vi "Instr_InitObject.vi"(8 "error in (no error)":errorcluster, 9 "Instrument Configuration":variant, 10 "GPIB address":string, 11 "KE236 in":refnum<class "KE236.lvclass">) -> (0 "error out":errorcluster, 3 "KE236 out":refnum<class "KE236.lvclass">)   [LabVIEW 2013, in "KE236.lvclass"]
uses:
  KE236.lvclass
  SupplyControl.lvclass
  InstrumentSetup.vi
  KE236_CommandsGlobal.vi
  InstrControl.lvclass
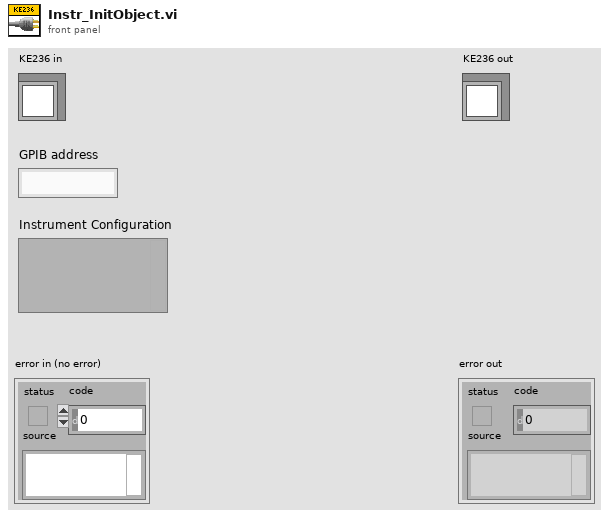
[diagram p1: front panel]
types:
  T1 = cluster{"current \ncompliance level":dbl, "compliance/\nmeasurement range (auto:0)":u16, "KE236":refnum<class "KE236.lvclass">}
  T2 = cluster{"Instrument name":string, "Command \"Reset\"":string, "Command \"Initialise\"":string, "Command \"Arm\"":string, "Command \"SetVolts\"":string, "Command \"Compliance?\"":string, "Command \"Standby\"":string, "Command \"Read Current\"":string}
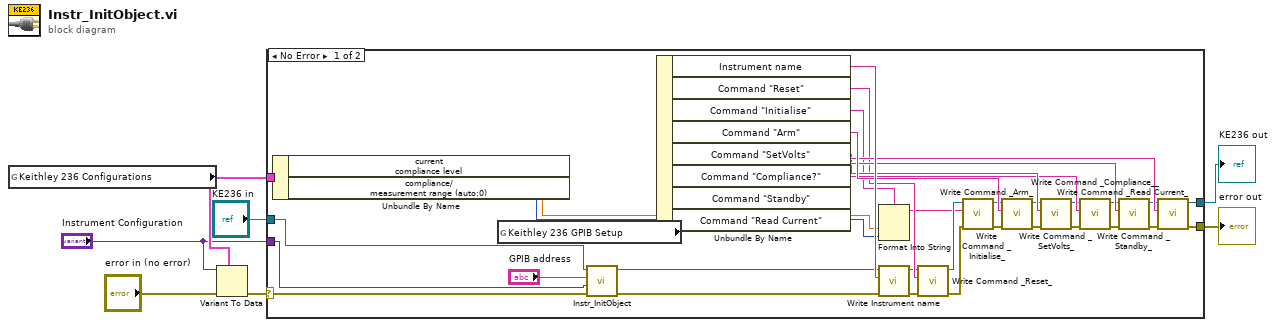
[diagram p0: block diagram]
diagram:
  n1 = global read "InstrumentSetup.vi" "Keithley 236 Configurations"() -> (w4:T1)
  n2 = Variant To Data(error in="error in (no error)", type=w4, Variant="Instrument Configuration") -> (error out=w2:errorcluster)  [unwired: 1 out]
  n3 = case shown="No Error" w2 {
    selector: w2 -> [w12 w44]
    tunnel: [w19 w44] -> w5
    tunnel: "KE236 in" -> [w14 w43]
    tunnel: [w20 w43] -> w6
    tunnel: w4 -> [w9 _]
    tunnel: "Instrument Configuration" -> [w8 _]
    frame No Error {
      n4 = Unbundle By Name(w9) -> ("current \ncompliance level"=w23:dbl, "compliance/\nmeasurement range (auto:0)"=w18:u16)
      n5 = global read "KE236_CommandsGlobal.vi" "Keithley 236 GPIB Setup"() -> (w17:T2)
      n6 = call-parent "Instr_InitObject.vi"("error in (no error)"=w12, "Instrument Configuration"=w8, "GPIB address"="GPIB address", "SupplyControl in"=w14) -> ("error out"=w11:errorcluster, "SupplyControl out"=w13:refnum<class "KE236.lvclass">)  [unwired: 6 in]
      n7 = Unbundle By Name(w17) -> ("Instrument name"=w42:string, "Command \"Reset\""=w36:string, "Command \"Initialise\""=w22:string, "Command \"Arm\""=w41:string, "Command \"SetVolts\""=w38:string, "Command \"Compliance?\""=w37:string, "Command \"Standby\""=w39:string, "Command \"Read Current\""=w40:string)
      n8 = Format Into String(format string=w22, w23, w18) -> (resulting string=w21:string)  [unwired: 2 in, 1 out]
      n9 = call-dynamic "Write Instrument name.vi"("error in (no error)"=w11, "Instrument name"=w42, "InstControl in"=w13) -> ("error out"=w15:errorcluster, "InstControl out"=w16:refnum<class "KE236.lvclass">)  [unwired: 7 in]
      n10 = call-dynamic "Write Command _Reset_.vi"("error in (no error)"=w15, "Command \"Reset\""=w36, "SupplyControl in"=w16) -> ("error out"=w29:errorcluster, "SupplyControl out"=w35:refnum<class "KE236.lvclass">)  [unwired: 7 in]
      n11 = call-dynamic "Write Command _Initialise_.vi"("error in (no error)"=w29, "Command \"Initialise\""=w21, "SupplyControl in"=w35) -> ("error out"=w28:errorcluster, "SupplyControl out"=w34:refnum<class "KE236.lvclass">)  [unwired: 7 in]
      n12 = call-dynamic "Write Command _Arm_.vi"("error in (no error)"=w28, "Command \"Arm\""=w41, "SupplyControl in"=w34) -> ("error out"=w27:errorcluster, "SupplyControl out"=w33:refnum<class "KE236.lvclass">)  [unwired: 7 in]
      n13 = call-dynamic "Write Command _SetVolts_.vi"("error in (no error)"=w27, "Command \"SetVolts\""=w38, "SupplyControl in"=w33) -> ("error out"=w26:errorcluster, "SupplyControl out"=w32:refnum<class "KE236.lvclass">)  [unwired: 7 in]
      n14 = call-dynamic "Write Command _Compliance__.vi"("error in (no error)"=w26, "Command \"Compliance?\""=w37, "SupplyControl in"=w32) -> ("error out"=w25:errorcluster, "SupplyControl out"=w31:refnum<class "KE236.lvclass">)  [unwired: 7 in]
      n15 = call-dynamic "Write Command _Standby_.vi"("error in (no error)"=w25, "Command \"Standby\""=w39, "SupplyControl in"=w31) -> ("error out"=w24:errorcluster, "SupplyControl out"=w30:refnum<class "KE236.lvclass">)  [unwired: 7 in]
      n16 = call-dynamic "Write Command _Read Current_.vi"("error in (no error)"=w24, "Command \"Read Current\""=w40, "SupplyControl in"=w30) -> ("error out"=w19:errorcluster, "SupplyControl out"=w20:refnum<class "KE236.lvclass">)  [unwired: 7 in]
    }
    frame Error {
    }
  }
  "error out" <- w5
  "KE236 out" <- w6
